vi "Convert String To Module And Assert Properties.vi"(7 "String in":string, 8 "error in (no error)":errorcluster, 9 "Slot Settings in":T2, 10 "Module Model in":T1, 11 "RSI Module Unit Tests in":refnum<class "RSI Module Unit Tests.lvclass">) -> (0 "error out":errorcluster, 2 "RSI Module out":refnum<class "RSI Module.lvclass">, 3 "RSI Module Unit Tests out":refnum<class "RSI Module Unit Tests.lvclass">)   [LabVIEW 2017, in "RSI Module Unit Tests.lvclass"]
uses:
  RSI Module Unit Tests.lvclass
  RSI Module/Slot Settings.ctl
  RSI Module/Module Models.ctl
  RSI Module/RSI Module.lvclass
  Modules.lvlib
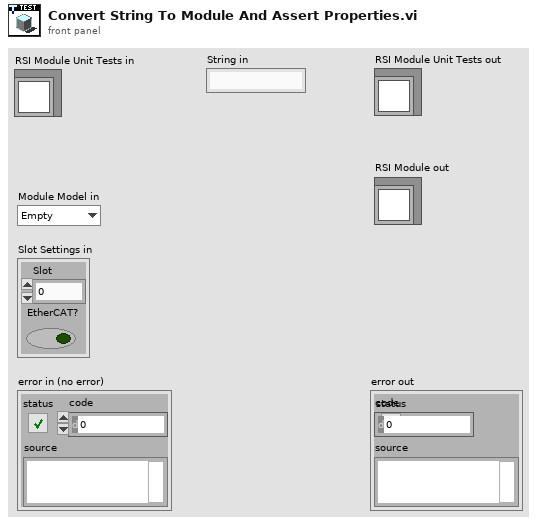
[diagram p1: front panel]
types:
  T1 = typedef "Modules.lvlib/RSI Module.lvclass/Module Models.ctl" = enum16{"Empty", "NI 9201", "NI 9203", "NI 9205", "NI 9206", "NI 9207", "NI 9208", "NI 9211", "NI 9212", "NI 9213", "NI 9214", "NI 9215", "NI 9217", "NI 9219", "NI 9220", "NI 9221", "NI 9222", "NI 9223", "NI 9225", "NI 9227", "NI 9229", "NI 9233", "NI 9234", "NI 9235", "NI 9236", "NI 9237", "NI 9239", "NI 9242", "NI 9244", "NI 9263", "NI 9264", "NI 9265", "NI 9266", "NI 9269", "NI 9375", "NI 9401", "NI 9402", "NI 9403", "NI 9411", "NI 9421", "NI 9422", "NI 9423", "NI 9425", "NI 9426", "NI 9435", "NI 9437", "NI 9472", "NI 9474", "NI 9475", "NI 9476", "NI 9477", "NI 9478", "NI 9481", "NI 9482", "NI 9485"}
  T2 = typedef "Modules.lvlib/RSI Module.lvclass/Slot Settings.ctl" = cluster{"Slot":u32, "EtherCAT?":bool}
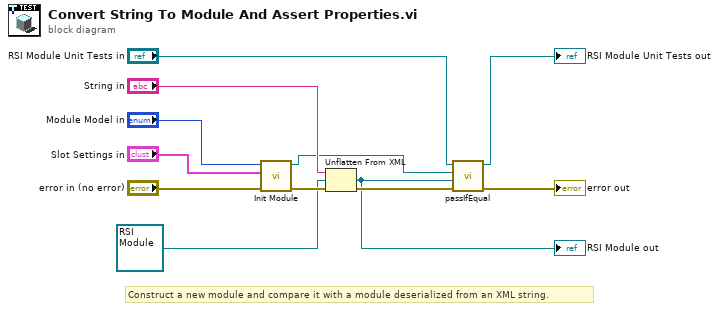
[diagram p0: block diagram]
diagram:
  # "Construct a new module and compare it with a module deserialized from an XML string."
  n1 = call "Init Module.vi"("error in (no error)"="error in (no error)", "Slot Settings"="Slot Settings in", "Module Model"="Module Model in") -> ("error out"=w7:errorcluster, "RSI Module out"=w8:refnum<class "RSI Module.lvclass">)  [unwired: 7 in]
  n2 = Unflatten From XML(xml string="String in", type=refnum<class "RSI Module.lvclass"> refnum ("Modules.lvlib:RSI Module.lvclass")) -> (value=w1:refnum<class "RSI Module.lvclass">)  [unwired: 1 in, 1 out]
  "RSI Module out" <- w1
  n3 = call-dynamic "passIfEqual.vi"("error in (no error)"=w7, "y"=w1, "x"=w8, "TestCase in"="RSI Module Unit Tests in") -> ("error out"=→"error out":errorcluster, "TestCase out"=→"RSI Module Unit Tests out":refnum<class "RSI Module Unit Tests.lvclass">)  [unwired: 6 in]
